vi "FTW-Collection-AddOrReplace-Variant.vi"(0 "Collection":refnum<class "FTW-Collection.lvclass">, 5 "Key":string, 7 "Value":variant, 11 "error in":errorcluster) -> (4 "Collection out":refnum<class "FTW-Collection.lvclass">, 6 "Replaced?":bool, 15 "error out":errorcluster)   [LabVIEW 2012, in "FTW-Collection.lvclass"]
uses:
  FTW-Collection.lvclass
  FTW-Collection.lvclass/FTW-Collection.ctl
panel:
  # "Inputs"
  # "Outputs"
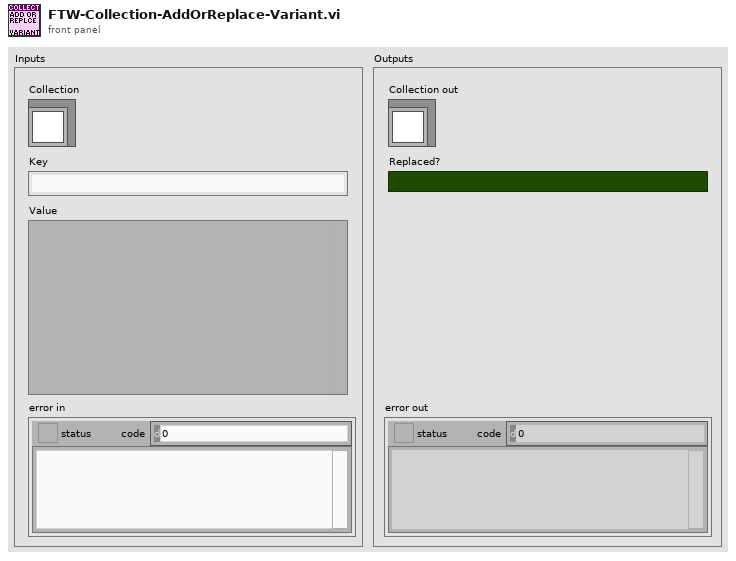
[diagram p1: front panel]
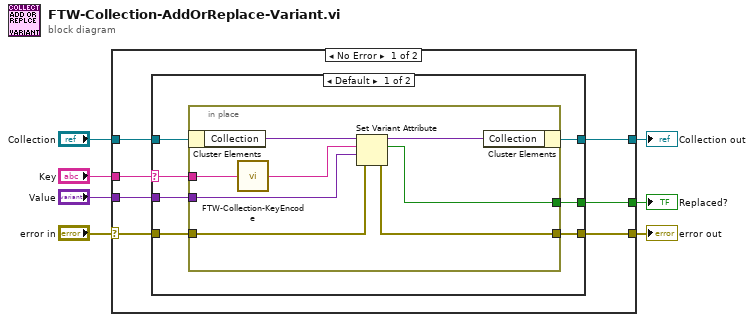
[diagram p0: block diagram]
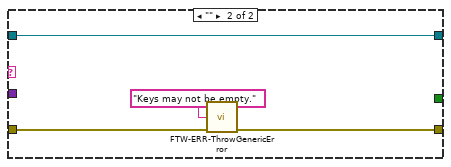
[diagram p2: hidden frame]
diagram:
  n1 = case shown="No Error" "error in" {
    selector: "error in" -> [w9 w35]
    tunnel: [w13 w35] -> w7
    tunnel: [w12 _] -> w5
    tunnel: "Collection" -> [w14 w34]
    tunnel: "Key" -> [w8 _]
    tunnel: [w11 w34] -> w2
    tunnel: "Value" -> [w10 _]
    frame No Error {
      n2 = case shown="Default" w8 {
        selector: w8 -> [w15 _]
        tunnel: w14 -> [w21 w33]
        tunnel: [w20 w31] -> w13
        tunnel: [w19 _] -> w12
        tunnel: [w18 w33] -> w11
        tunnel: w10 -> [w17 _]
        tunnel: w9 -> [w16 w32]
        frame Default {
          n3 = in-place {
            in-place-border: w15 -> [w27]
            in-place-border: w16 -> [w26]
            in-place-border: [w25] -> w20
            in-place-border: [w24] -> w19
            in-place-border: w17 -> [w23]
            n4 = in-place-cluster #1(w21) -> ("Collection"=w29:variant)
            n5 = call "FTW-Collection-KeyEncode.vi"("Key"=w27) -> ("Encoded Key"=w22:string)
            n6 = Set Variant Attribute(Variant=w29, name=w22, value=w23, error in=w26) -> (Variant out=w28:variant, replaced=w24:bool, error out=w25:errorcluster)
            n7 = in-place-cluster #1("Collection"=w28) -> (w18:refnum<class "FTW-Collection.lvclass">)
          }
        }
        frame "" {
          n8 = call "FTW-ERR-ThrowGenericError.vi"("Error Message"="Keys may not be empty.", "error in"=w32) -> ("error out"=w31:errorcluster)  [unwired: 13 in]
        }
      }
    }
    frame Error {
    }
  }
  "error out" <- w7
  "Replaced?" <- w5
  "Collection out" <- w2
